vi "Initialize.vi"(8 "error in":errorcluster, 11 "TSI 3085 Nano in":refnum<class "TSI 3085 Nano.lvclass">) -> (0 "error out":errorcluster, 3 "TSI 3085 Nano out":refnum<class "TSI 3085 Nano.lvclass">)   [LabVIEW 2014, in "TSI 3085 Nano.lvclass"]
uses:
  TSI 3085 Nano.lvclass
  DMA.lvclass/DMA.ctl
  Accessors/Write ri.vi
  Accessors/Write ro.vi
  Accessors/Write Leff.vi
  DMA.lvclass
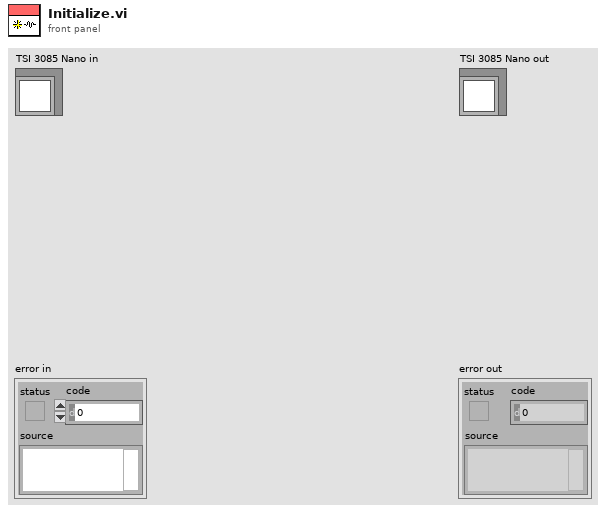
[diagram p1: front panel]
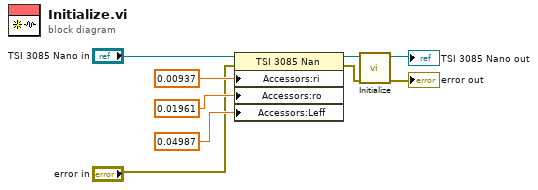
[diagram p0: block diagram]
diagram:
  n1 = property class="TSI 3085 Nan"(reference="TSI 3085 Nano in", error in="error in", "Accessors:ri"=0.00937 ("ri"), "Accessors:ro"=0.01961 ("ro"), "Accessors:Leff"=0.04987 ("Leff")) -> (reference out=w9:refnum<class "TSI 3085 Nano.lvclass">, error out=w5:errorcluster)
  n2 = call-parent "Initialize.vi"("error in"=w5, "DMA in"=w9) -> ("error out"=→"error out":errorcluster, "DMA out"=→"TSI 3085 Nano out":refnum<class "TSI 3085 Nano.lvclass">)  [unwired: 8 in]
